vi "Write AI.Channels.vi"(8 "error in (no error)":errorcluster, 10 "AI.Channels":T1, 11 "DAQ in":refnum<class "DAQ.lvclass">) -> (0 "error out":errorcluster, 3 "DAQ out":refnum<class "DAQ.lvclass">)   [LabVIEW 2016, in "DAQ.lvclass"]
uses:
  DAQ.lvclass
  Typedefs/PrivateEvents--DAQ.AI.Channels.ctl
  DAQ.lvclass/DAQ.ctl
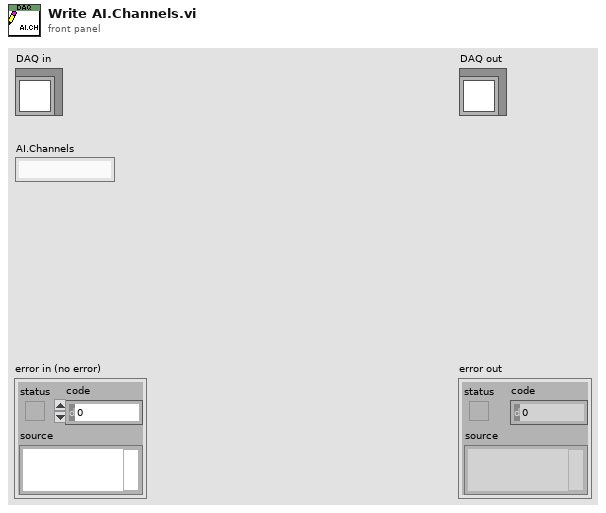
[diagram p1: front panel]
types:
  T1 = typedef "DAQ.lvclass/PrivateEvents--DAQ.AI.Channels.ctl" = string
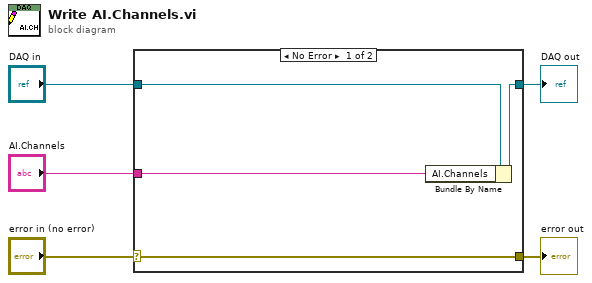
[diagram p0: block diagram]
diagram:
  n1 = case shown="No Error" "error in (no error)" {
    selector: "error in (no error)" -> [w9 w10]
    tunnel: [w9 w10] -> w4
    tunnel: [w7 w11] -> w2
    tunnel: "DAQ in" -> [w8 w11]
    tunnel: "AI.Channels" -> [w6 _]
    frame No Error {
      n2 = Bundle By Name(cluster=w8, "AI.Channels"=w6) -> (w7:refnum<class "DAQ.lvclass">)
    }
    frame Error {
    }
  }
  "error out" <- w4
  "DAQ out" <- w2
